vi "Save Recall Setup.vi"(8 "Error In (no error)":errorcluster, 9 "Mode (T: Save)":bool=TRUE, 10 "Buffer (1: Buffer 1)":u16(ring)=1 items=["None", "Buffer 1", "Buffer 2", "Buffer 3", "Buffer 4", "Buffer 5", "Buffer 6", "Buffer 7", "Buffer 8", "Buffer 9"], 11 "VISA Resource Name":refnum<visa-resource-name>) -> (0 "Error Out":errorcluster, 3 "VISA Resource Name Out":refnum<visa-resource-name>)   [LabVIEW 2010, in "Stanford Research 844.lvlib"]
doc: "This VI saves and recalls instrument's setup."
uses:
  <instrlib>/Stanford Research 844/Stanford Research 844.lvlib
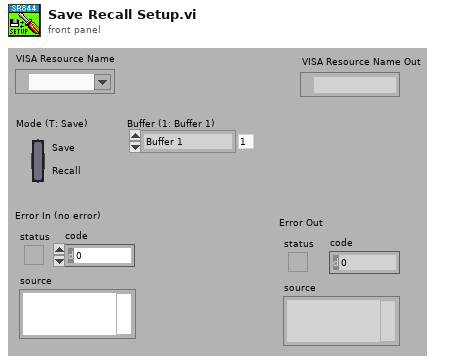
[diagram p1: front panel]
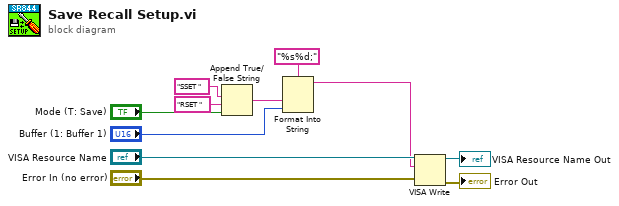
[diagram p0: block diagram]
diagram:
  n1 = Append True/False String(1:"Mode (T: Save)", 2:"RSET " ("false string"), 3:"SSET " ("true string")) -> (0:w3:string)  [unwired: 1 in]
  n2 = Format Into String(format string="%s%d;", w3, "Buffer (1: Buffer 1)") -> (resulting string=w1:string)  [unwired: 2 in, 1 out]
  n3 = VISA Write(VISA resource name="VISA Resource Name", write buffer=w1, error in (no error)="Error In (no error)") -> (VISA resource name out=→"VISA Resource Name Out":refnum<visa-resource-name>, error out=→"Error Out":errorcluster)  [unwired: 1 out]
